vi "str to uint8.vi"(2 "String":string) -> (6 "uint8":u8)   [LabVIEW 2013, in "CreateOPCUAServerAuto.lvlib"]
uses:
  CreateOPCUAServerAuto.lvlib
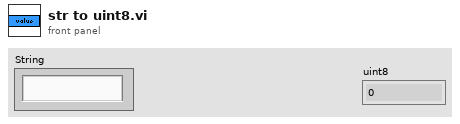
[diagram p1: front panel]
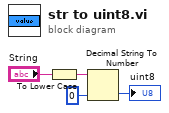
[diagram p0: block diagram]
diagram:
  n1 = To Lower Case(string="String") -> (all lower case string=w3:string)
  n2 = Decimal String To Number(string=w3, default (0L)=u8 0 ("default (0 I32)")) -> (number=→"uint8":u8)  [unwired: 1 in, 1 out]
